vi "SRV_Dialogs for System Config Selection.vi"(0 "System Config Names":string[](array[string])) -> (6 "System Config Name":string, 8 "Cancelled?":bool, 10 "New?":bool)   [LabVIEW 2009]
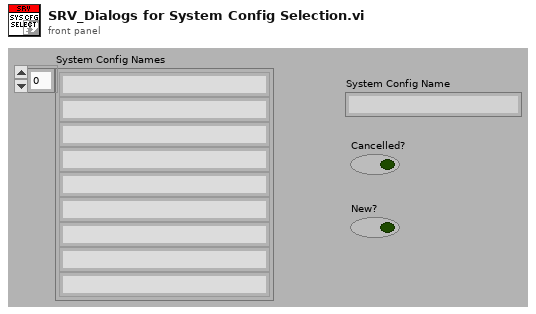
[diagram p1: front panel]
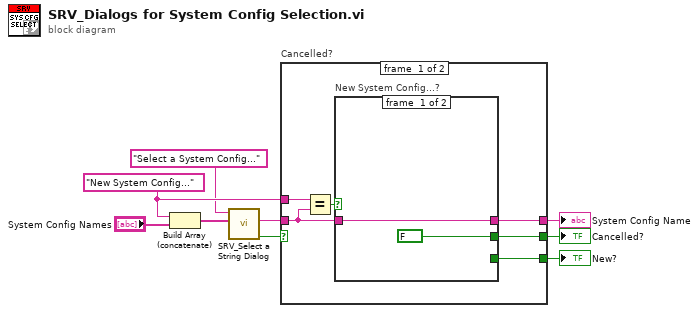
[diagram p0: block diagram]
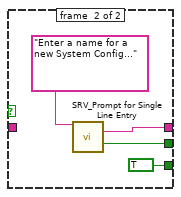
[diagram p2: hidden frame]
diagram:
  w6 = "New System Config..."
  n1 = Build Array (concatenate)(w6, "System Config Names") -> (w3:string[])
  n2 = call "SRV_Select a String Dialog.vi"("String List"=w3, "Prompt (Select one item.)"="Select a System Config...") -> ("Cancelled?"=w4:bool, "Selected String"=w5:string)  [unwired: 8 in]
  n3 = case "Cancelled?" shown="False" w4 {
    selector: w4 -> [_ w22]
    tunnel: w5 -> [w13 _]
    tunnel: [w12 w22] -> w7
    tunnel: w6 -> [w15 _]
    tunnel: [w11 _] -> w8
    tunnel: [w10 _] -> w9
    frame #0 {
      n4 = Equal?(x=w15, y=w13) -> (x = y?=w14:bool)
      n5 = case "New System Config...?" shown="True" w14 {
        tunnel: w13 -> [w16 _]
        tunnel: [FALSE ("Canceled") w20] -> w12
        tunnel: [w16 w19] -> w11
        tunnel: [_ TRUE ("New?")] -> w10
        frame #0 {
        }
        frame #1 {
          n6 = call "SRV_Prompt for Single Line Entry.vi"("Prompt"="Enter a name for a new System Config...") -> ("Entered String"=w19:string, "Canceled"=w20:bool)  [unwired: 12 in, 1 out]
        }
      }
    }
    frame #1 {
    }
  }
  "New?" <- w9
  "System Config Name" <- w8
  "Cancelled?" <- w7
